vi "Get Old Tweets - Continuous.vi"() -> ()   [LabVIEW 2011]
doc: "This example gets old tweets. The first time Get Old Tweets.vi runs, it grabs the tweets starting from the top of the user's timeline. The following runs to Get Old Tweets.vi will get tweets older then the oldest mentions from the previous run."
uses:
  Controls/Tweet.ctl
  i3-twitter.lvlib
panel:
  out "Tweets":T1[](array[typedef])
  in  "stop":bool
  out "Time Stamp of Oldest Tweet":timestamp
  in  "Screen Name (Empty)":string
  out "Num of Tweets Read":i32
  in  "Num of Tweets to Read":i32
  in  "Consumer Key":string
  in  "Consumer Secret":string
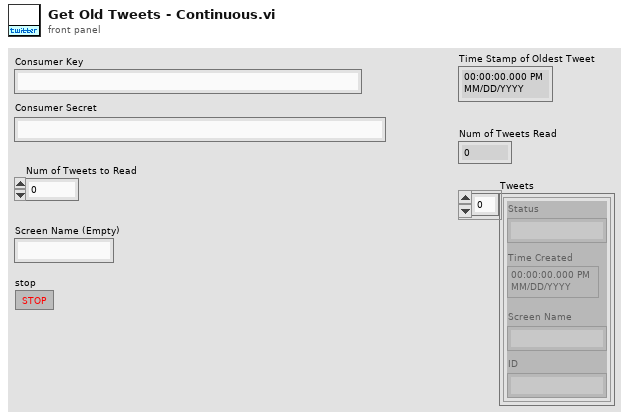
[diagram p1: front panel]
types:
  T1 = typedef "i3-twitter.lvlib/Tweet.ctl" = cluster{"Status":string, "Time Created":timestamp, "Screen Name":string, "ID":string}
  T2 = typedef "i3-twitter.lvlib/Twitter Handle.ctl" = cluster{"OAuth Credentials":T3, "since ID":string, "max ID":string, "Screen Name":string}
  T3 = typedef "i3-oauth.lvlib/OAuth Credentials.ctl" = cluster{"Consumer Key":string, "Signature Method":T4, "Token":string, "Version":string, "Token Secret":string, "Consumer Secret":string}
  T4 = typedef "i3-oauth.lvlib/Signature Method.ctl" = enum16{"HMAC-MD5", "HMAC-SHA1", "HMAC-SHA224", "HMAC-SHA256", "HMAC-SHA384", "HMAC-SHA512"}
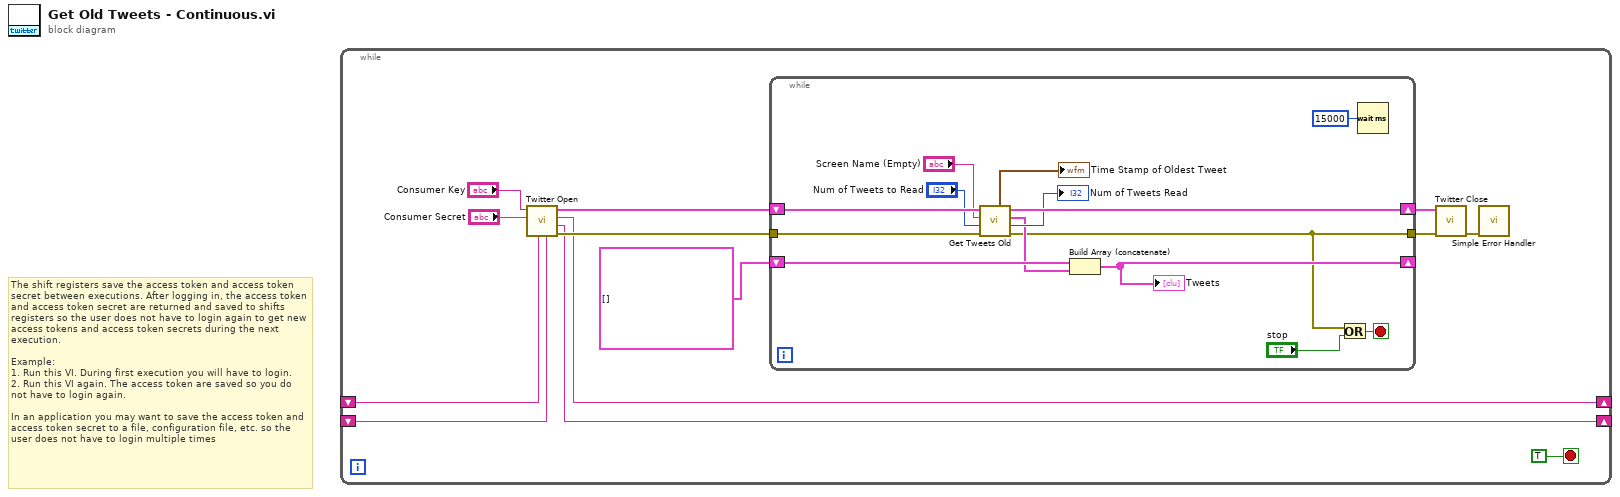
[diagram p0: block diagram]
diagram:
  # "The shift registers save the access token and access token secret between executions. After logging in, the access token and access token secret are returned and saved to shifts registers so the user does not have to login again to get new access tokens and access token secrets during the next execution.\n\nExample:\n1. Run this VI. During first execution you will have to login.\n2. Run this VI again. The access token are saved so you do not have to login again.\n\nIn an application you may want to save the access token and access token secret to a file, configuration file, etc. so the user does not have to login multiple times"
  n1 = while {
    shift-right: [w1] -> _
    shift-left: _ -> [w4]
    shift-right: [w2] -> _
    shift-left: _ -> [w3]
    stop <- TRUE stop-if-true
    n2 = call "Twitter Open.vi"("Access Token Secret (In)"=w3, "Access Token (In)"=w4, "Consumer Secret"="Consumer Secret", "Consumer Key"="Consumer Key") -> ("error out"=w7:errorcluster, "Access Token Secret (Out)"=w2:string, "Access Token (Out)"=w1:string, "Twitter Handle Out"=w11:T2)  [unwired: 4 in]
    n3 = while {
      tunnel: w7 -> [w26]
      tunnel: [w18] -> w10
      shift-right: [w25] -> w9
      shift-left: w11 -> [w27]
      shift-right: [w23] -> _
      shift-left: T1[] [] ("Tweets Array") -> [w22]
      stop <- w17 stop-if-true
      n4 = call "Get Tweets Old.vi"("error in"=w26, "Tweets to Read (10)"="Num of Tweets to Read", "Screen Name (Empty)"="Screen Name (Empty)", "Twitter Handle In"=w27) -> ("error out"=w18:errorcluster, "Actual Num of Tweets Read"=→"Num of Tweets Read":i32, "Old Tweets Read"=w20:T1[], "Twitter Handle Out"=w25:T2, "Time Stamp of Oldest Tweet"=→"Time Stamp of Oldest Tweet":timestamp)  [unwired: 3 in]
      n5 = Build Array (concatenate)(w22, w20) -> (w23:T1[])
      "Tweets" <- w23
      n6 = Or(x=w18, y="stop") -> (x .or. y?=w17:bool)
      n7 = Wait (ms)(milliseconds to wait=u32 15000) -> ()  [unwired: 1 out]
    }
    n8 = call "Twitter Close.vi"("error in"=w10, "Twitter Handle In"=w9) -> ("error in"=w5:errorcluster)  [unwired: 9 in]
    n9 = call <vilib>:"Simple Error Handler.vi"("error in (no error)"=w5) -> ()  [unwired: 4 in, 5 out]
  }
